vi "Status Page GUID.vi"() -> (3 "Status GUID":string="565c4ee4-8051-44d7-8930-f003aae83434")   [LabVIEW 2020, in "DSF Shared.lvlib"]
uses:
  DSF Shared.lvlib
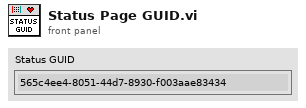
[diagram p1: front panel]
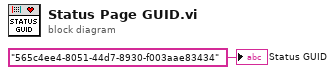
[diagram p0: block diagram]
diagram:
  "Status GUID" <- "565c4ee4-8051-44d7-8930-f003aae83434" ("Data Sharing Framework")
